vi "Get Interface.vi"(8 "error in (no error)":errorcluster, 11 "index":i32) -> (0 "error out":errorcluster, 2 "lvwpcap_interface_array":string[](array[string]))   [LabVIEW 2017, in "lvwpcap.lvlib"]
uses:
  lvwpcap.lvlib
  LVpcap.dll
panel:
  # "Select Help»Show Context Help and move the cursor over the VI icon to display help for this VI."
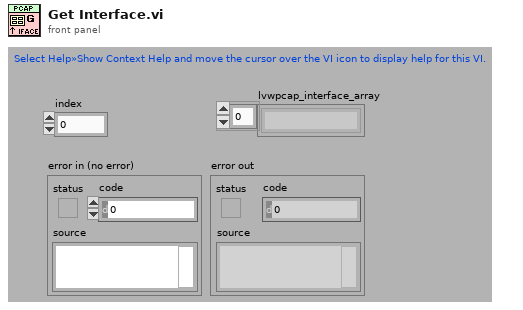
[diagram p1: front panel]
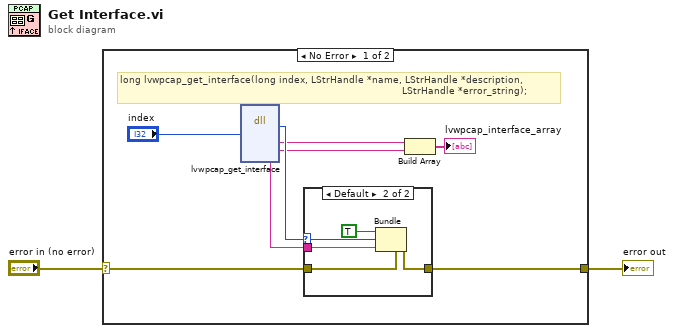
[diagram p0: block diagram]
diagram:
  n1 = case shown="No Error" "error in (no error)" {
    selector: "error in (no error)" -> [w3 w17]
    tunnel: [w9 w17] -> w2
    frame No Error {
      # "long lvwpcap_get_interface(long index, LStrHandle *name, LStrHandle *description,\n                                                                                              LStrHandle *error_string);"
      n2 = dll-call lib="C:/Users/Michaello/Desktop/MGR NOWEEEEEEEEEEEEEE/MR PROFINET 2017/Lib/WinPcap/LVpcap.dll" fn="lvwpcap_get_interface"("index"="index") -> ("return type"=w8:i32, "name"=w6:string, "description"=w5:string, "error_string"=w7:string)  [unwired: 7 in, 2 out]
      n3 = case shown="Default" w8 {
        selector: w8 -> [_ w15]
        tunnel: w7 -> [_ w14]
        tunnel: w3 -> [w11 w16]
        tunnel: [w11 w12] -> w9
        frame 0 {
        }
        frame Default {
          n4 = Bundle(cluster=w16, "status"=TRUE, "code"=w15, "source"=w14) -> (w12:errorcluster)
        }
      }
      n5 = Build Array(w6, w5) -> (→"lvwpcap_interface_array":string[])
    }
    frame Error {
    }
  }
  "error out" <- w2
